vi "SystemPraefix.vi"(8 "Fehler (Eingang)":errorcluster) -> (0 "Fehler (Ausgang)":errorcluster, 3 "SystemPraefix":string)   [LabVIEW 2020, in "allgemeine Sub-VIs.lvlib"]
uses:
  allgemeine Sub-VIs.lvlib
  Seiten/System Einstellungen V2/Aktioen FGV System Konstanten.ctl
  Seiten/System Einstellungen V2/System Einstellungen V2.lvlib
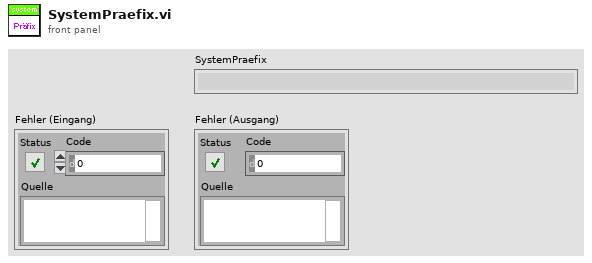
[diagram p1: front panel]
types:
  T1 = typedef "System Einstellungen V2.lvlib/Aktioen FGV System Konstanten.ctl" = enum16{"lesen", "laden", "speichern", "Sprache"}
  T2 = cluster{"Modell":string, "ProjektNummer":string, "Software Version":string, "Seriennummer":string}
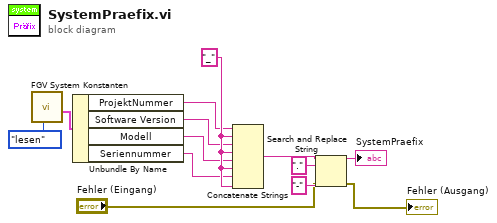
[diagram p0: block diagram]
diagram:
  w12 = "_"
  n1 = call "FGV System Konstanten.vi"("Aktionen"=Aktioen_FGV_System_Konstanten."lesen") -> ("Cluster out"=w6:T2)  [unwired: 6 in, 4 out]
  n2 = Unbundle By Name(w6) -> ("ProjektNummer"=w7:string, "Software Version"=w5:string, "Modell"=w4:string, "Seriennummer"=w3:string)
  n3 = Concatenate Strings(w7, w12, w5, w12, w4, w12, w3, w12) -> (w11:string)
  n4 = Search and Replace String(input string=w11, search string="." ("Such-String"), replace string="-" ("Ersetzungs-String (\"\")"), error in="Fehler (Eingang)") -> (result string=→"SystemPraefix":string, error out=→"Fehler (Ausgang)":errorcluster)  [unwired: 4 in, 2 out]
